vi "Example.vi"   [LabVIEW 2014]
uses:
  Config Data.lvclass
  Config Data.lvclass/Config Data.ctl
  <vilib>/Utility/config.llb/Read Key (Boolean).vi
  <userlib>/_Session Fwk/Session - Root.lvclass
  <vilib>/Utility/config.llb/NI_LVConfig.lvlib
types:
  T1 = typedef "Session - Root.lvclass/Session Handle.ctl" = refnum<data-value>
  T2 = typedef "NI_LVConfig.lvlib/Config Data RefNum.ctl" = refnum<k1>
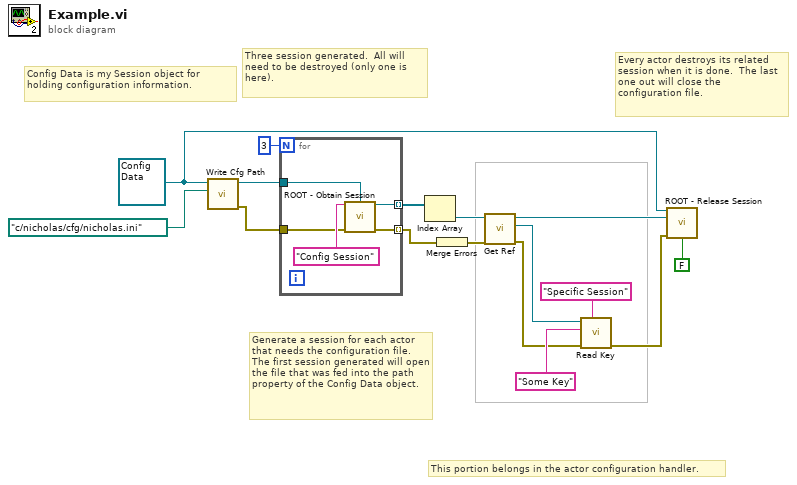
[diagram p0: block diagram]
diagram:
  w5 = refnum<class "Config Data.lvclass"> refnum ("Config Data")
  # "Three session generated.  All will need to be destroyed (only one is here)."
  # "Config Data is my Session object for holding configuration information."
  # "Generate a session for each actor that needs the configuration file.  The first session generated will open the file that was fed into the path property of the Config Data object."
  # "This portion belongs in the actor configuration handler."
  # "Every actor destroys its related session when it is done.  The last one out will close the configuration file."
  n1 = call "Write Cfg Path.vi"("Cfg Path"=path "c:/nicholas/cfg/nicholas.ini", "Config Data in"=w5) -> ("error out"=w8:errorcluster, "Config Data out"=w15:refnum<class "Config Data.lvclass">)  [unwired: 8 in]
  n2 = for {
    N: 3 -> [_]
    tunnel: w15 -> [w21]
    tunnel: [w19] -> w14 mode=indexing
    tunnel: w8 -> [w18]
    tunnel: [w17] -> w7 mode=indexing
    n3 = call <userlib>:"ROOT - Obtain Session.vi"("Session Name ()"="Config Session", "OBJ - Session"=w21, "error in (no error)"=w18) -> ("Session Handle"=w19:T1, "error out"=w17:errorcluster)  [unwired: 10 in, 1 out]
  }
  n4 = Index Array(array=w14) -> (element=w13:T1)  [unwired: 1 in]
  n5 = Merge Errors(w7) -> (w6:errorcluster)
  n6 = call "Get Ref.vi"("error in (no error)"=w6, "Session Handle In"=w13) -> ("error out"=w9:errorcluster, "Ref"=w12:T2, "Session Handle Out"=w4:T1)  [unwired: 7 in]
  n7 = call-poly <vilib>:"Read Key.vi"("section"="Specific Session", "error in (no error)"=w9, "key"="Some Key", "refnum"=w12) -> ("error out"=w3:errorcluster)  [unwired: 4 in, 3 out]
  n8 = call <userlib>:"ROOT - Release Session.vi"("OBJ - Session in"=w5, "Session Handle in"=w4, "error in (no error)"=w3, "force destroy? (F)"=FALSE) -> ()  [unwired: 9 in, 3 out]
